vi "Configure Synchronization Timeout.vi"(0 "VISA resource name":refnum<visa-resource-name>, 5 "Synchronization Timeout (0 s)":dbl format="%#.6f", 11 "error in (no error)":errorcluster) -> (4 "VISA resource name out":refnum<visa-resource-name>, 15 "error out":errorcluster)   [LabVIEW 2012, in "NH Research Regenerative Test Series.lvlib"]
doc: "This sets the synchronization timeout. The timeout is from receiving to executing a command or measurement. This allows multiple modules to receive commands sequentially but execute simultaneously using hardware synchronization signals. Set to 0 there is no synchronization. Greater than 0, the module will wait up to this time for other modules to process commands and operate in sync. Reset is 0, range is 0 to 0.5 second."
uses:
  <instrlib>/NH Research Regenerative Test Series/NH Research Regenerative Test Series.lvlib
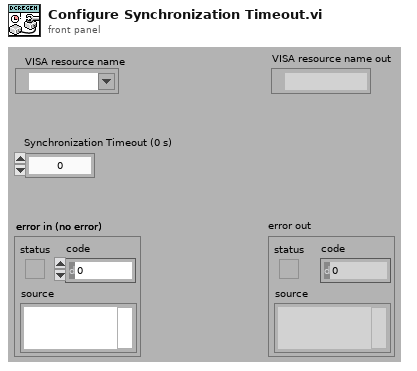
[diagram p1: front panel]
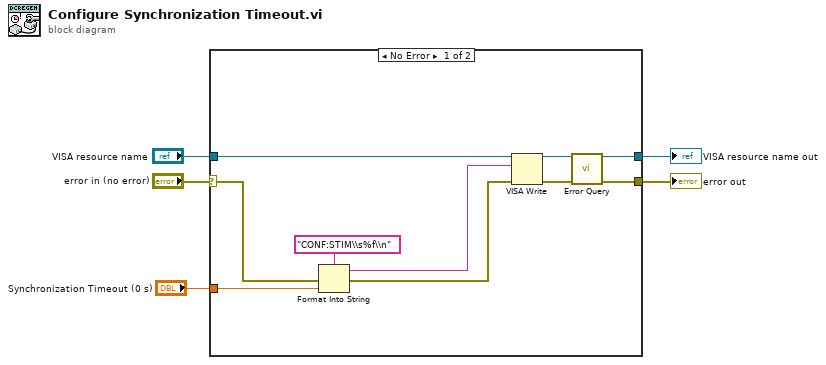
[diagram p0: block diagram]
diagram:
  n1 = case shown="No Error" "error in (no error)" {
    selector: "error in (no error)" -> [w9 w17]
    tunnel: "VISA resource name" -> [w15 w16]
    tunnel: [w14 w16] -> w4
    tunnel: [w13 w17] -> w3
    tunnel: "Synchronization Timeout (0 s)" -> [w10 _]
    frame No Error {
      n2 = Format Into String(format string="CONF:STIM\\s%f\\n", error in=w9, w10) -> (resulting string=w7:string, error out=w8:errorcluster)  [unwired: 1 in]
      n3 = VISA Write(VISA resource name=w15, write buffer=w7, error in (no error)=w8) -> (VISA resource name out=w12:refnum<visa-resource-name>, error out=w11:errorcluster)  [unwired: 1 out]
      n4 = call <instrlib>:"Error Query.vi"("VISA resource name"=w12, "error in (no error)"=w11) -> ("VISA resource name out"=w14:refnum<visa-resource-name>, "error out"=w13:errorcluster)  [unwired: 10 in, 2 out]
    }
    frame Error {
    }
  }
  "error out" <- w3
  "VISA resource name out" <- w4
